vi "disable_and_gray_out_buttons.vi"(10 "Disabled":T1(ring)=enum."Disabled and Grayed Out", 11 "Array":refnum<vi>[](array[refnum])) -> ()   [LabVIEW 2017]
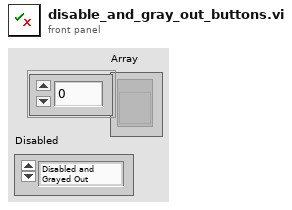
[diagram p1: front panel]
types:
  T1 = enum8{"Enabled", "Disabled", "Disabled and Grayed Out"}
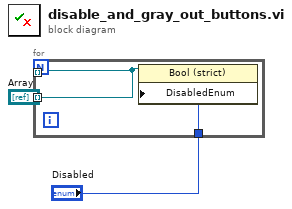
[diagram p0: block diagram]
diagram:
  n1 = for {
    tunnel: [w4] -> _ mode=indexing
    tunnel: "Array" -> [w4] mode=indexing
    tunnel: "Disabled" -> [w3]
    n2 = property on="Property Node" class="Bool (strict)"(reference=w4, "DisabledEnum"=w3) -> ()  [unwired: 1 in, 2 out]
  }
